vi "Module - Button Strip.vi"() -> ()   [LabVIEW 2020]
uses:
  Control/Button Strip.ctl
  Control/State - Button Strip.ctl
  Control/State - eFGV.ctl
panel:
  in  "Radio Buttons":T1
  out "error out":errorcluster
  in  "error in (no error)":errorcluster
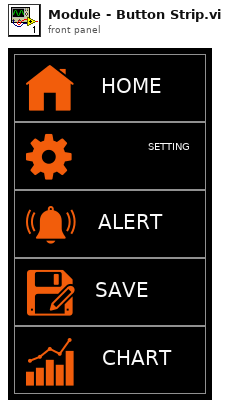
[diagram p1: front panel]
types:
  T1 = typedef "Button Strip.ctl" = enum32{"Home", "Setting", "Alert", "Save", "Chart"}
  T2 = typedef "State - Button Strip.ctl" = enum16{"Init module", "Register event", "Idle", "Send Event", "Unregister event", "Close module"}
  T3 = typedef "State - eFGV.ctl" = enum16{"Init", "Read", "Write", "Close"}
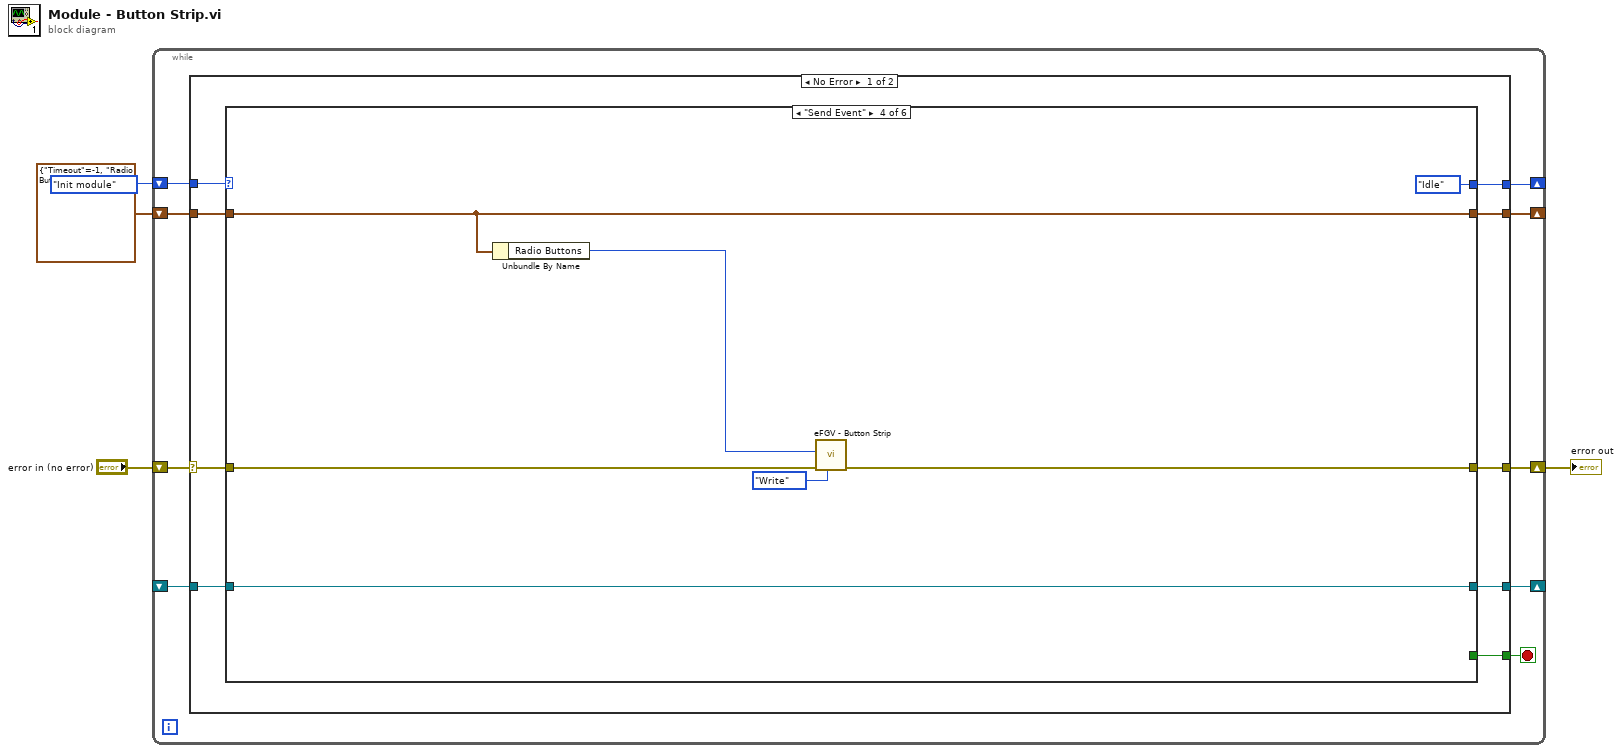
[diagram p0: block diagram]
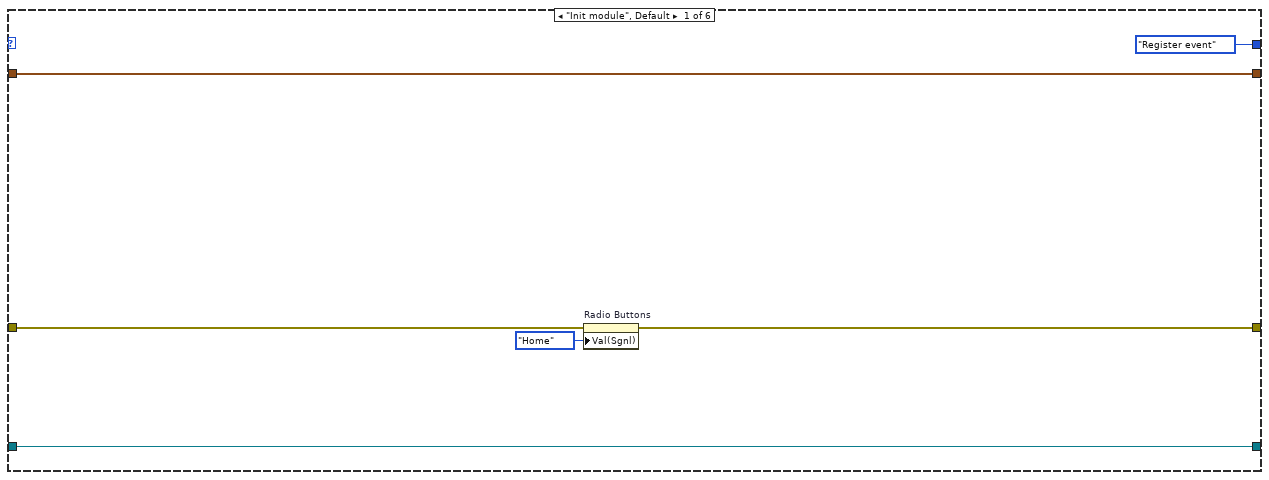
[diagram p2: hidden frame]
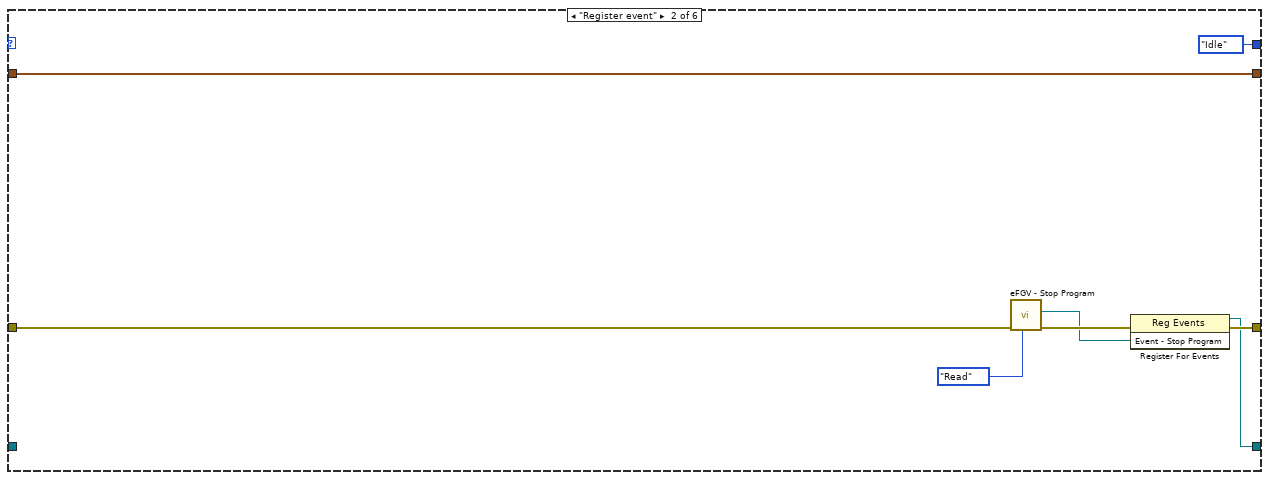
[diagram p3: hidden frame]
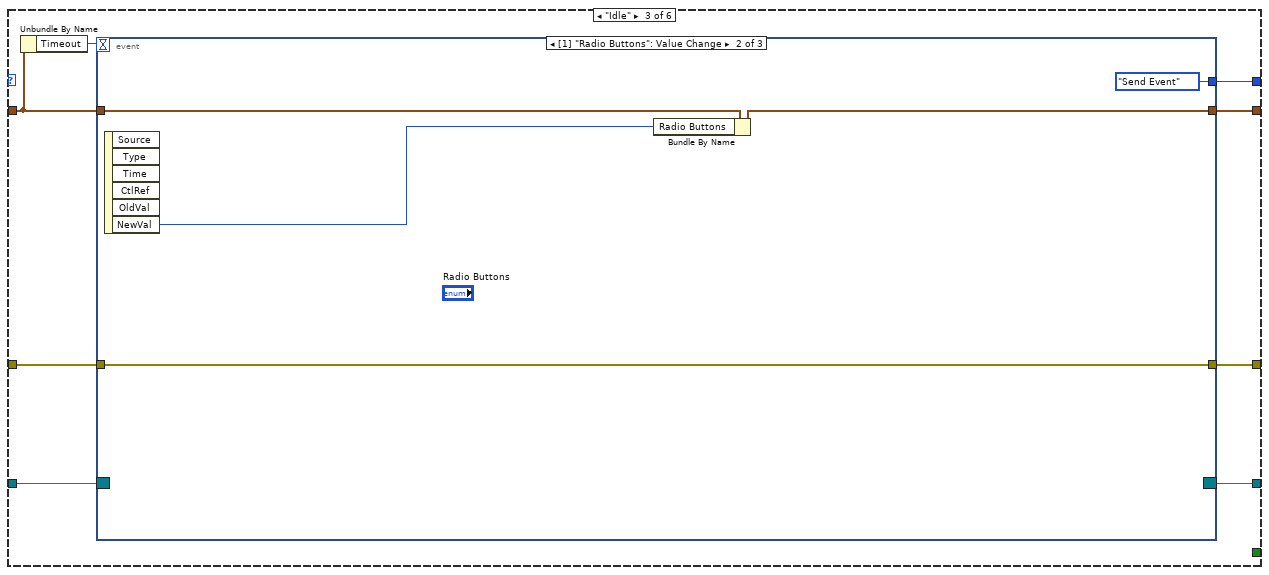
[diagram p4: hidden frame]
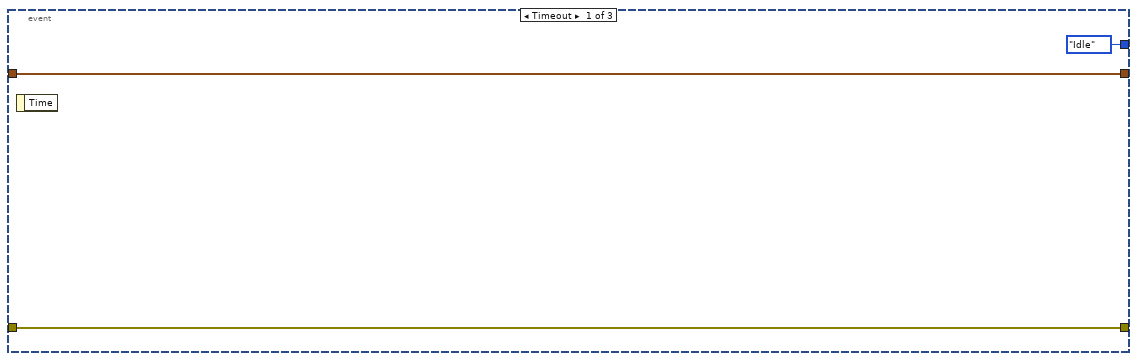
[diagram p5: hidden frame]
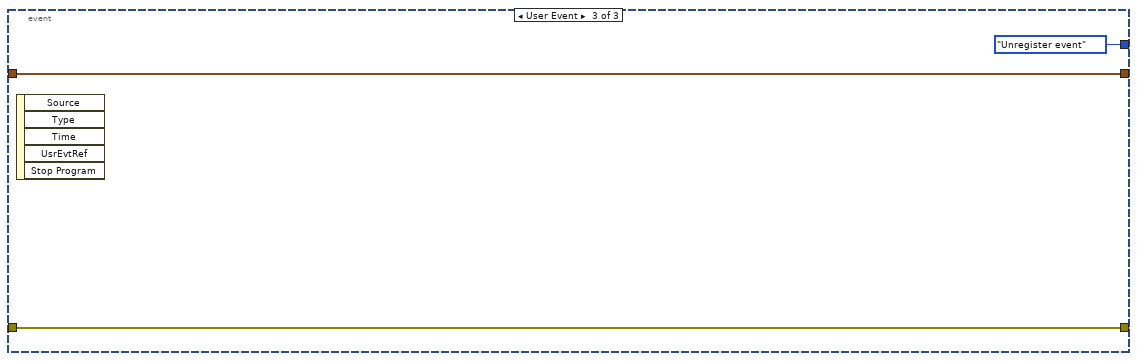
[diagram p6: hidden frame]
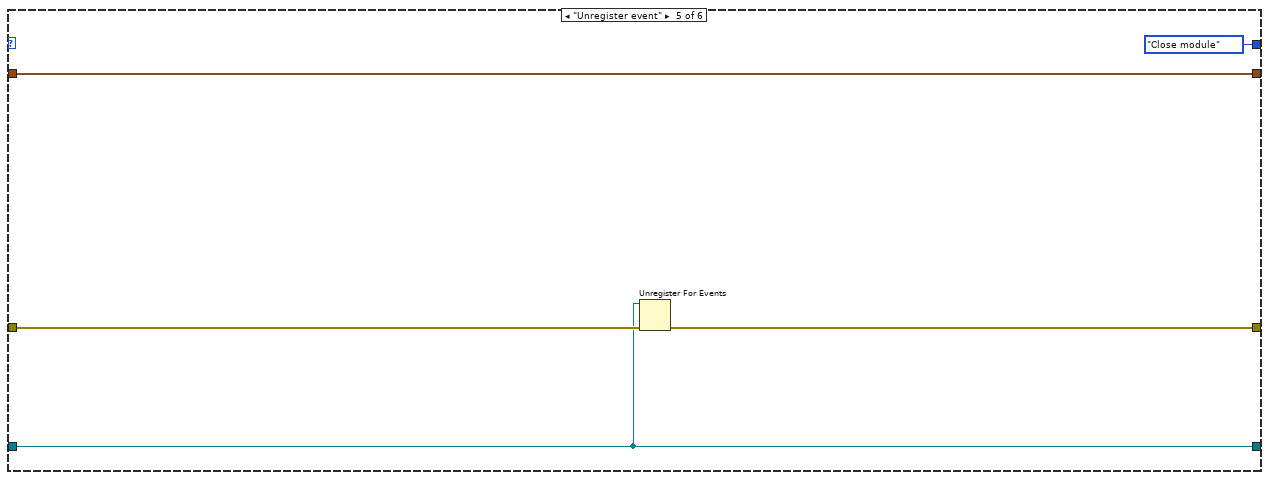
[diagram p7: hidden frame]
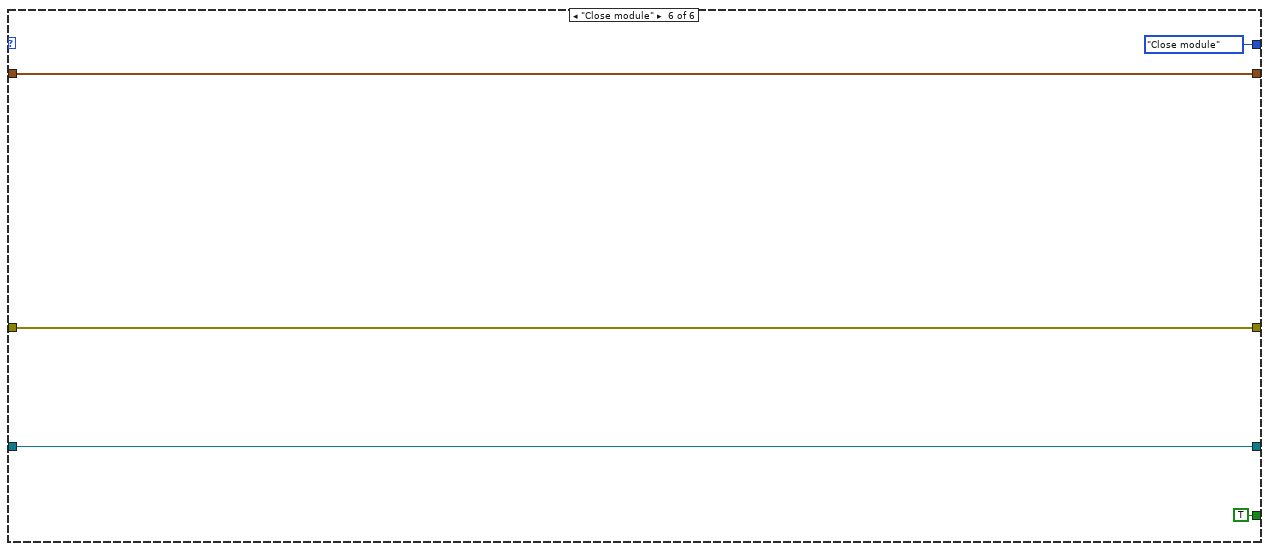
[diagram p8: hidden frame]
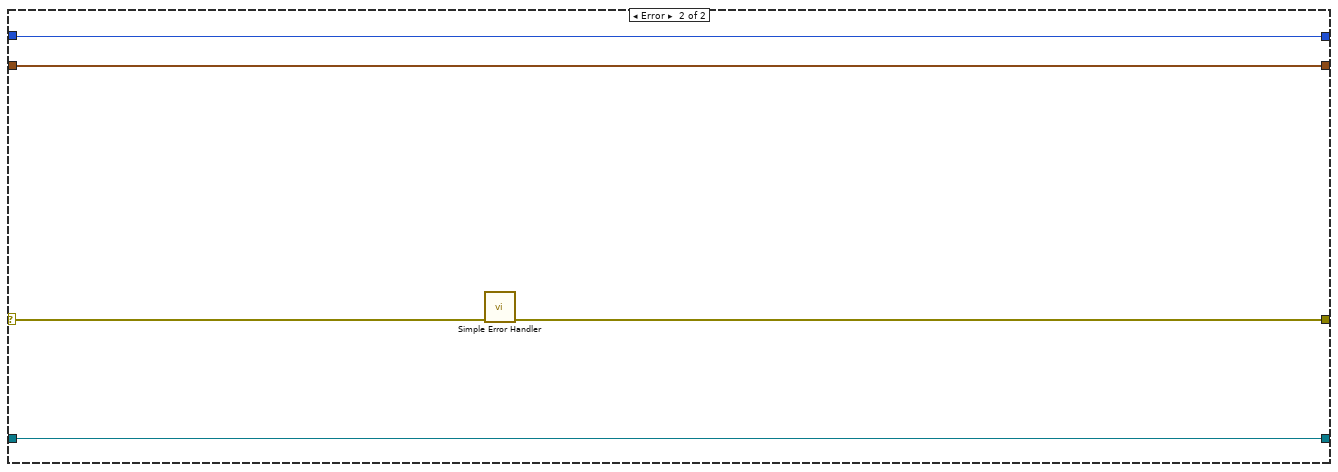
[diagram p9: hidden frame]
diagram:
  n1 = while {
    shift-right: [w11] -> w3
    shift-left: "error in (no error)" -> [w13]
    shift-right: [w5] -> _
    shift-left: State_-_Button_Strip."Init module" -> [w12]
    shift-right: [w10] -> _
    shift-left: _ -> [w9]
    shift-right: [w7] -> _
    shift-left: cluster{"Timeout":i32, "Radio Buttons":T1} {"Timeout"=-1, "Radio Buttons"=enum."Setting"} -> [w8]
    stop <- w6 stop-if-true
    n2 = case shown="No Error" w13 {
      selector: w13 -> [w21 w77]
      tunnel: w12 -> [w22 w73]
      tunnel: [w20 w76] -> w11
      tunnel: [w19 w75] -> w10
      tunnel: w9 -> [w18 w75]
      tunnel: w8 -> [w17 w74]
      tunnel: [w16 w74] -> w7
      tunnel: [w15 _] -> w6
      tunnel: [w14 w73] -> w5
      frame No Error {
        n3 = case shown="\"Send Event\"" w22 {
          tunnel: w21 -> [w25 w32 w41 w60 w66 w72]
          tunnel: [w24 w36 w38 w59 w65 w72] -> w20
          tunnel: [w28 w35 w39 w62 w64 w71] -> w19
          tunnel: w18 -> [w28 _ w40 w62 w64 w71]
          tunnel: w17 -> [w27 w34 w43 w61 w67 w70]
          tunnel: [w27 w34 w42 w61 w67 w70] -> w16
          tunnel: [_ _ _ _ _ TRUE] -> w15
          tunnel: [State_-_Button_Strip."Register event" State_-_Button_Strip."Idle" w37 State_-_Button_Strip."Idle" State_-_Button_Strip."Close module" State_-_Button_Strip."Close module"] -> w14
          frame "Init module", Default {
            n4 = property on="Radio Buttons" class="RadioBtnsControl (strict)"(error in=w25, "Val(Sgnl)"=Button_Strip."Home" ("Value (Signaling)")) -> (error out=w24:errorcluster)  [unwired: 1 in, 1 out]
          }
          frame "Register event" {
            n5 = call "eFGV - Stop Program.vi"("State - eFGV"=State_-_eFGV."Read", "error in (no error)"=w32) -> ("error out"=w33:errorcluster, "Event - Stop Program"=w31:refnum<user-event>)  [unwired: 8 in]
            n6 = register-events(error in=w33, w31) -> (reference out=w35:refnum<event-registration>, error out=w36:errorcluster)  [unwired: 1 in]
          }
          frame "Idle" {
            n7 = Unbundle By Name(w43) -> ("Timeout"=w44:i32)
            n8 = event shown="[1] \"Radio Buttons\": Value Change" {
              selector: w40 -> [_ _ _]
              dyn-events: [_ _ _] -> w39
              timeout: w44 -> [_ _ _]
              tunnel: w43 -> [w47 w52 w55]
              tunnel: [w47 w49 w55] -> w42
              tunnel: w41 -> [w46 w50 w53]
              tunnel: [w46 w50 w53] -> w38
              tunnel: [State_-_Button_Strip."Idle" State_-_Button_Strip."Send Event" State_-_Button_Strip."Unregister event"] -> w37
              event Timeout {
                n9 = event-data() -> ()  [unwired: 1 in, 1 out]
              }
              event Value Change {
                n10 = event-data() -> ("NewVal"=w48:T1)  [unwired: 1 in, 5 out]
                n11 = Bundle By Name(cluster=w52, "Radio Buttons"=w48) -> (w49:cluster{"Timeout":i32, "Radio Buttons":T1})
              }
              event User Event {
                n12 = event-data() -> ()  [unwired: 1 in, 5 out]
              }
            }
          }
          frame "Send Event" {
            n13 = Unbundle By Name(w61) -> ("Radio Buttons"=w57:T1)
            n14 = call "eFGV - Button Strip.vi"("State - eFGV"=State_-_eFGV."Write", "error in (no error)"=w60, "Radio Buttons"=w57) -> ("error out"=w59:errorcluster)  [unwired: 7 in, 1 out]
          }
          frame "Unregister event" {
            n15 = Unregister For Events(event registration refnum=w64, error in=w66) -> (error out=w65:errorcluster)
          }
          frame "Close module" {
          }
        }
      }
      frame Error {
        n16 = call <vilib>:"Simple Error Handler.vi"("error in (no error)"=w77) -> ("error out"=w76:errorcluster)  [unwired: 4 in, 4 out]
      }
    }
  }
  "error out" <- w3
